vi "nirviSatArithSubtEmu(unsigned).vi"(2 "y":u16, 3 "x":u16) -> (0 "overflow":bool, 1 "x-y":u16)   [LabVIEW 2017]
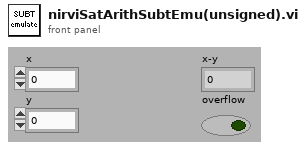
[diagram p1: front panel]
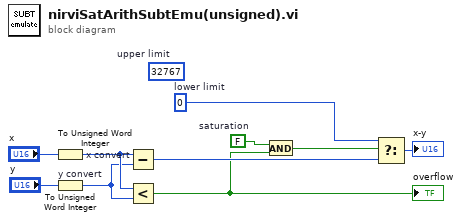
[diagram p0: block diagram]
diagram:
  w1 = u16 0  # lower limit
  (unwired) u16 32767  # upper limit
  w9 = FALSE  # saturation
  n1 = To Unsigned Word Integer "x convert"(number="x") -> (unsigned 16bit integer=w4:u16)
  n2 = To Unsigned Word Integer "y convert"(number="y") -> (unsigned 16bit integer=w3:u16)
  n3 = Subtract(x=w4, y=w3) -> (x-y=w8:u16)
  n4 = Less?(x=w4, y=w3) -> (x < y?=w2:bool)
  "overflow" <- w2
  n5 = And(x=w9, y=w2) -> (x .and. y?=w10:bool)
  n6 = Select(t=w1, s=w10, f=w8) -> (s? t:f=→"x-y":u16)
